vi "SmartDrive.vi"(6 "Aim-Assist":bool, 7 "Throttle Correction":bool, 8 "Aim-Assist Gain":dbl, 10 "Turn":dbl, 11 "Power":dbl) -> (2 "Magnitude Right":dbl, 3 "Magnitude Left":dbl)   [LabVIEW 2017]
uses:
  <vilib>/Rock Robotics/Network Tables/NT Read Number.vi
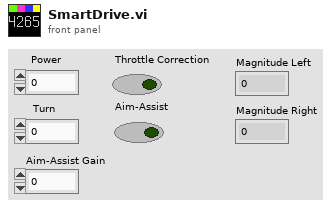
[diagram p1: front panel]
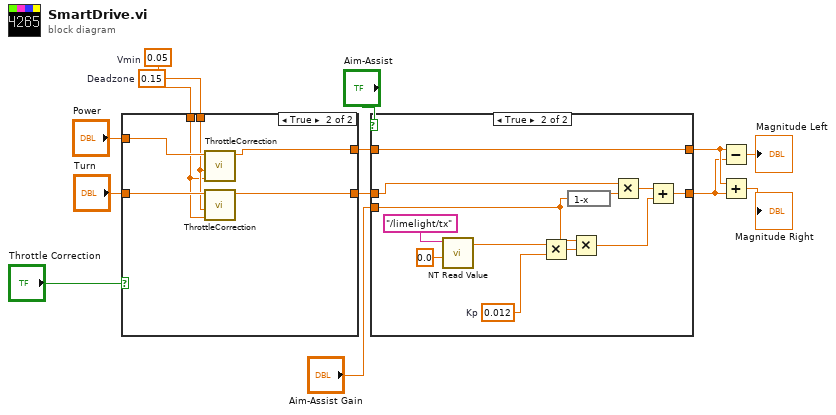
[diagram p0: block diagram]
diagram:
  w9 = 0.05  # Vmin
  w10 = 0.15  # Deadzone
  n1 = case shown="True" "Throttle Correction" {
    tunnel: "Power" -> [w15 w21]
    tunnel: "Turn" -> [w14 w20]
    tunnel: w10 -> [_ w19]
    tunnel: w9 -> [_ w18]
    tunnel: [w15 w17] -> w4
    tunnel: [w14 w16] -> w3
    frame False {
    }
    frame True {
      n2 = call "ThrottleCorrection.vi"("Vmin"=w18, "Deadzone"=w19, "Input"=w21) -> ("Output"=w17:dbl)  [unwired: 8 in]
      n3 = call "ThrottleCorrection.vi"("Vmin"=w18, "Deadzone"=w19, "Input"=w20) -> ("Output"=w16:dbl)  [unwired: 8 in]
    }
  }
  n4 = case shown="True" "Aim-Assist" {
    tunnel: [w23 w35] -> w5
    tunnel: w4 -> [w23 w35]
    tunnel: w3 -> [w22 w28]
    tunnel: [w22 w30] -> w2
    tunnel: "Aim-Assist Gain" -> [_ w25]
    frame False {
    }
    frame True {
      w32 = 0.012  # Kp
      n5 = call-poly <vilib>:"NT Read Value.vi"("Default Value"=0.0, "Name"="/limelight/tx") -> ("Numeric"=w31:dbl)  [unwired: 8 in, 1 out]
      n6 = Multiply(x=w31, y=w32) -> (x*y=w26:dbl)
      n7 = expression code="1-x"(w25) -> (w27:dbl)
      n8 = Multiply(x=w25, y=w26) -> (x*y=w24:dbl)
      n9 = Multiply(x=w28, y=w27) -> (x*y=w29:dbl)
      n10 = Add(x=w29, y=w24) -> (x+y=w30:dbl)
    }
  }
  n11 = Subtract(x=w5, y=w2) -> (x-y=→"Magnitude Left":dbl)
  n12 = Add(x=w5, y=w2) -> (x+y=→"Magnitude Right":dbl)
